vi "Read Instrument code names.vi"(1 "Measurement Setup File":string) -> (0 "List of Code Names":string[](array[string]))   [LabVIEW 2022 SP3]
uses:
  File/Setup_Filetype.ctl
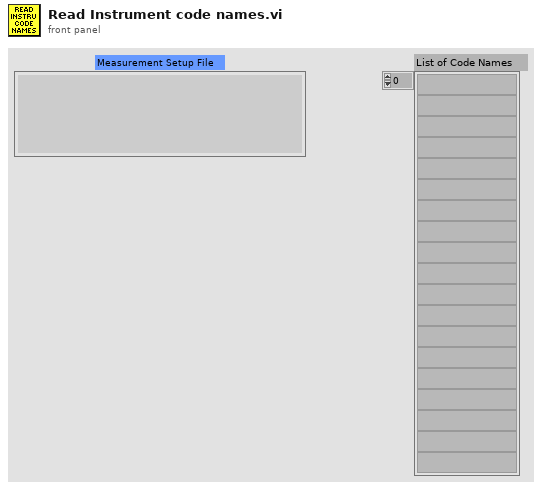
[diagram p1: front panel]
types:
  T1 = typedef "Setup_Filetype.ctl" = enum16{"Measurement Setups", "Calibration Setups", "General", "Results File Plotter Setups", "Speed Calib Tweaks"}
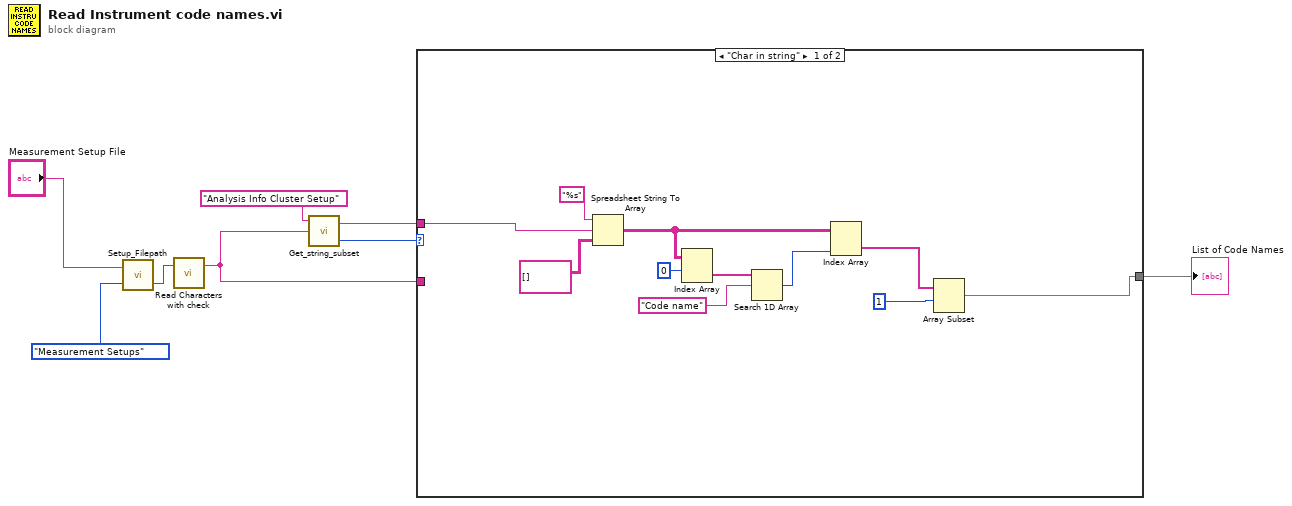
[diagram p0: block diagram]
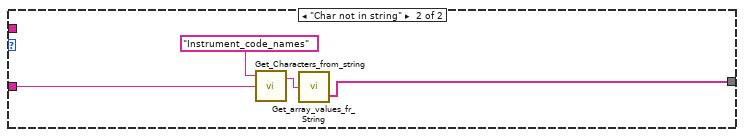
[diagram p2: hidden frame]
diagram:
  n1 = call "Setup_Filepath.vi"("Setup File Type"=Setup_Filetype."Measurement Setups", "Filename in"="Measurement Setup File") -> ("Filename Out"=w1:path)  [unwired: 1 out]
  n2 = call "Read Characters with check.vi"("file (use dialog)"=w1) -> ("Read String"=w2:string)  [unwired: 1 in, 1 out]
  n3 = call "Get_string_subset.vi"("String to split"=w2, "File Label"="Analysis Info Cluster Setup") -> ("Status"=w7:enum16{"Char in string", "Char not in string"}, "Output string"=w3:string)  [unwired: 2 in]
  n4 = case shown="\"Char in string\"" w7 {
    tunnel: w2 -> [_ w21]
    tunnel: [w10 w20] -> w4
    tunnel: w3 -> [w9 _]
    frame "Char in string" {
      n5 = Spreadsheet String To Array(format string="%s", spreadsheet string=w9, array type (2D Dbl)=string[][] []) -> (array=w14:string[][])  [unwired: 1 in]
      n6 = Index Array(array=w14, index (row)=0) -> (element=w19:string[])  [unwired: 1 in]
      n7 = Search 1D Array(1D array=w19, element="Code name") -> (index of element=w13:i32)  [unwired: 1 out]
      n8 = Index Array(array=w14, index (col)=w13) -> (element=w12:string[])  [unwired: 1 in]
      n9 = Array Subset(array=w12, index=1) -> (w10:string[])  [unwired: 1 in]
    }
    frame "Char not in string" {
      n10 = call "Get_Characters_from_string.vi"("Input string"=w21, "Variable name"="Instrument_code_names" ("Label for characters")) -> ("Value"=w23:string)  [unwired: 1 in, 1 out]
      n11 = call "Get_array_values_fr_String.vi"("String Value"=w23) -> ("String array"=w20:string[])  [unwired: 1 out]
    }
  }
  "List of Code Names" <- w4
